vi "VGap_GapIncrease.vi"(1 "error in (no error)":errorcluster, 2 "Step Increase (um)":i32, 3 "Gap Increase (um)":i32, 4 "System Index In":u32) -> (0 "error out":errorcluster)   [LabVIEW 2010]
panel:
  out "Current Step":i32
  out "Number of Step":dbl
  out "Position 3":dbl
  out "Position 2":dbl
  out "Position 1":dbl
  out "Initial Position 1 (um) 3":dbl
  out "Initial Position 1 (um) 2":dbl
  out "Initial Position 1 (um)":dbl
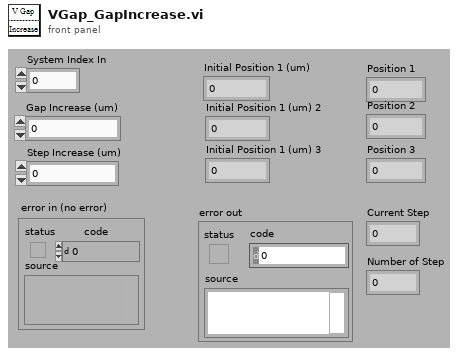
[diagram p1: front panel]
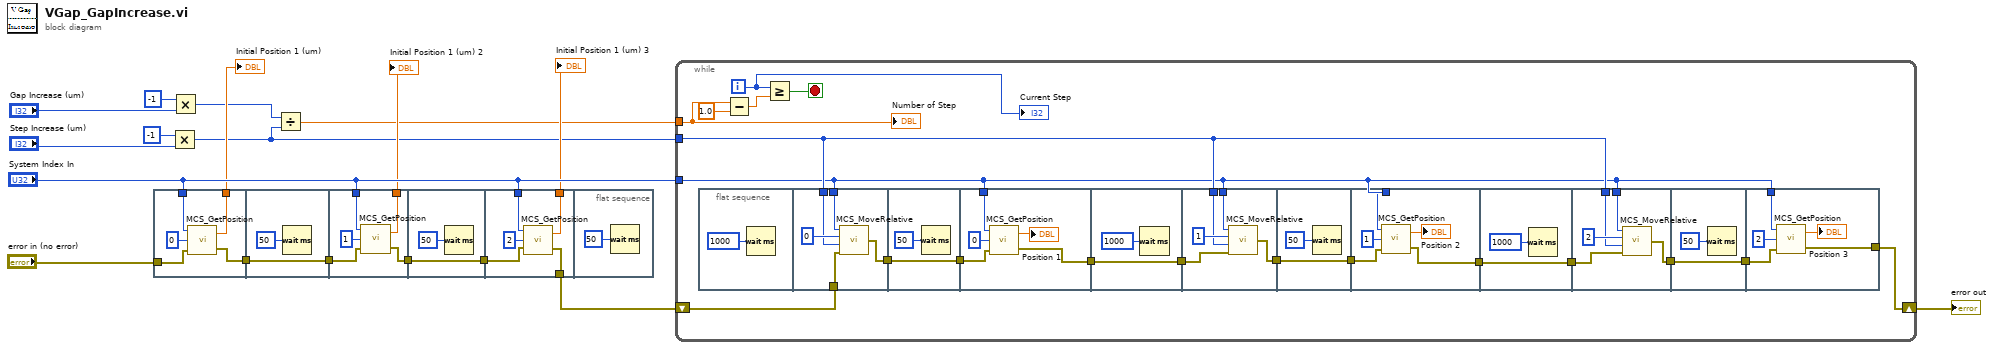
[diagram p0: block diagram]
diagram:
  n1 = flat-sequence {
    tunnel: "System Index In" -> [w22]
    tunnel: [w21] -> w17
    tunnel: [w20] -> w3
    tunnel: "error in (no error)" -> [w19]
    tunnel: [w24] -> w4
    tunnel: w3 -> [w24]
    tunnel: "System Index In" -> [w29]
    tunnel: [w28] -> w16
    tunnel: [w27] -> w5
    tunnel: w4 -> [w26]
    tunnel: [w31] -> w6
    tunnel: w5 -> [w31]
    tunnel: "System Index In" -> [w36]
    tunnel: [w35] -> w15
    tunnel: [w34] -> w7
    tunnel: w6 -> [w33]
    frame #0 {
      n2 = call "MCS_GetPosition.vi"("error in (no error)"=w19, "Channel Index In"=u32 0, "System Index In"=w22) -> ("error out"=w20:errorcluster, "Position (um)"=w21:dbl)
    }
    frame #1 {
      n3 = Wait (ms)(milliseconds to wait=u32 50) -> ()  [unwired: 1 out]
    }
    frame #2 {
      n4 = call "MCS_GetPosition.vi"("error in (no error)"=w26, "Channel Index In"=u32 1, "System Index In"=w29) -> ("error out"=w27:errorcluster, "Position (um)"=w28:dbl)
    }
    frame #3 {
      n5 = Wait (ms)(milliseconds to wait=u32 50) -> ()  [unwired: 1 out]
    }
    frame #4 {
      n6 = call "MCS_GetPosition.vi"("error in (no error)"=w33, "Channel Index In"=u32 2, "System Index In"=w36) -> ("error out"=w34:errorcluster, "Position (um)"=w35:dbl)
    }
    frame #5 {
      n7 = Wait (ms)(milliseconds to wait=u32 50) -> ()  [unwired: 1 out]
    }
  }
  n8 = Multiply(x=-1, y="Step Increase (um)") -> (x*y=w8:i32)
  n9 = Multiply(x=-1, y="Gap Increase (um)") -> (x*y=w10:i32)
  n10 = Divide(x=w10, y=w8) -> (x/y=w9:dbl)
  n11 = while {
    tunnel: "System Index In" -> [w55]
    tunnel: w9 -> [w40]
    tunnel: w8 -> [w56]
    shift-right: [w54] -> w1
    shift-left: w7 -> [w53]
    i -> [w42]
    stop <- w57 stop-if-true
    n12 = flat-sequence {
      tunnel: w55 -> [w63]
      tunnel: w56 -> [w61]
      tunnel: w53 -> [w60]
      tunnel: [w59] -> w51
      tunnel: [w64] -> w52
      tunnel: w51 -> [w64]
      tunnel: w55 -> [w69]
      tunnel: w52 -> [w67]
      tunnel: [w66] -> w49
      tunnel: [w71] -> w50
      tunnel: w49 -> [w71]
      tunnel: w55 -> [w76]
      tunnel: w56 -> [w75]
      tunnel: w50 -> [w74]
      tunnel: [w73] -> w47
      tunnel: [w78] -> w48
      tunnel: w47 -> [w78]
      tunnel: w55 -> [w83]
      tunnel: w48 -> [w81]
      tunnel: [w80] -> w45
      tunnel: [w85] -> w46
      tunnel: w45 -> [w85]
      tunnel: w55 -> [w90]
      tunnel: w56 -> [w89]
      tunnel: w46 -> [w88]
      tunnel: [w87] -> w43
      tunnel: [w92] -> w44
      tunnel: w43 -> [w92]
      tunnel: w55 -> [w97]
      tunnel: [w95] -> w54
      tunnel: w44 -> [w94]
      frame #0 {
        n13 = Wait (ms)(milliseconds to wait=u32 1000) -> ()  [unwired: 1 out]
      }
      frame #1 {
        n14 = call "MCS_MoveRelative.vi"("error in (no error)"=w60, "Moving Distance (um)"=w61, "Channel Index In"=u32 0, "System Index In"=w63) -> ("error out"=w59:errorcluster)
      }
      frame #2 {
        n15 = Wait (ms)(milliseconds to wait=u32 50) -> ()  [unwired: 1 out]
      }
      frame #3 {
        n16 = call "MCS_GetPosition.vi"("error in (no error)"=w67, "Channel Index In"=u32 0, "System Index In"=w69) -> ("error out"=w66:errorcluster, "Position (um)"=→"Position 1":dbl)
      }
      frame #4 {
        n17 = Wait (ms)(milliseconds to wait=u32 1000) -> ()  [unwired: 1 out]
      }
      frame #5 {
        n18 = call "MCS_MoveRelative.vi"("error in (no error)"=w74, "Moving Distance (um)"=w75, "Channel Index In"=u32 1, "System Index In"=w76) -> ("error out"=w73:errorcluster)
      }
      frame #6 {
        n19 = Wait (ms)(milliseconds to wait=u32 50) -> ()  [unwired: 1 out]
      }
      frame #7 {
        n20 = call "MCS_GetPosition.vi"("error in (no error)"=w81, "Channel Index In"=u32 1, "System Index In"=w83) -> ("error out"=w80:errorcluster, "Position (um)"=→"Position 2":dbl)
      }
      frame #8 {
        n21 = Wait (ms)(milliseconds to wait=u32 1000) -> ()  [unwired: 1 out]
      }
      frame #9 {
        n22 = call "MCS_MoveRelative.vi"("error in (no error)"=w88, "Moving Distance (um)"=w89, "Channel Index In"=u32 2, "System Index In"=w90) -> ("error out"=w87:errorcluster)
      }
      frame #10 {
        n23 = Wait (ms)(milliseconds to wait=u32 50) -> ()  [unwired: 1 out]
      }
      frame #11 {
        n24 = call "MCS_GetPosition.vi"("error in (no error)"=w94, "Channel Index In"=u32 2, "System Index In"=w97) -> ("error out"=w95:errorcluster, "Position (um)"=→"Position 3":dbl)
      }
    }
    n25 = Subtract(x=w40, y=1.0) -> (x-y=w41:dbl)
    n26 = Greater Or Equal?(x=w42, y=w41) -> (x >= y?=w57:bool)
    "Number of Step" <- w40
    "Current Step" <- w42
  }
  "error out" <- w1
  "Initial Position 1 (um)" <- w17
  "Initial Position 1 (um) 2" <- w16
  "Initial Position 1 (um) 3" <- w15
